vi "HFRR ADV v024 new software.vi"() -> ()   [LabVIEW 2025] (continued)
-:"], ["Ch-Heater:", "НАГРЕВ:"], ["Ch-Humidity Wet:", "CH-Увлажнение:"], ["Ch-Humidity Dry:", "CH-Осушение:"], ["Heater On", "НАГРЕВ ВКЛ"], ["Heater Off", "НАГРЕВ ВЫКЛ"], ["On", "ВКЛ"], ["Off", "ВЫКЛ"], ["TEXT REPORT", "ПРОТОКОЛ ИСПЫТАНИЯ"], ["Open Data File", "ОТКРЫТЬ ФАЙЛ ДАННЫХ"], ["Refresh", "ОБНОВЛЕНО"], ["Tittle", "заглавие"], ["Sample Design", "Образец"], ["Tested date", "Дата"], ["Sample ID ", "Имя образца"], ["Tested by", "Испытано"], ["System Configured Printers ", "Сконфигурированные принтеры"], ["Selected Printer", "Выбранный принтер"], ["Select Printer 3", "Выбрать  Печать"], ["Print", "Печать"], [":-@(WINDUCOM : RECIPROCATORY TEST RIG    DEFINITON FILE )      ", "(Анализатор HFRR с возвратно-поступательным механизмом для определения смазывающей способности дизельных топлив )"], ["Tested by:", "Оператор:"], ["          TIME;      COF;       STROKE  (mm);     AIR TEMP ( Deg C);  TEMP ( Deg C);  HUMIDITY ( Rh );", "КОЭФФИЦИЕНТ ТРЕНИЯ;   Инсульт; ТЕМПЕРАТУРА ВОЗДУХА; ВЛАЖНОСТЬ;"], ["Export", "Экспорт"], ["Temperature Intercept :", "ТЕМП перехват:"], ["Air Temperature Intercept:", "ТЕМП  ВОЗДУХА перехват:"], ["Select File Type ", "Выберете формат файла"], ["S.NO", "S.NO"], ["Trip", ""]]
  out "Residual Uno":string
  out "Residual Due":string
  out "String":string="C:\\Winducom 2010\\1582\\1582\\"
  out "file path":path=path "C:/Windows/wndcm_pw_stdED hfrr.txt"
  out "string":string="49\r50\r51\r10"
  out "x = y?":bool
  out "dipl pwd":string="@143$\n"
  out "string1 4":string
  out "string1 3":string
  out "string1 2":string
  out "string1":string
  out "stopT":bool
  out "Elapsed time 3":dbl=0.10620016403198242 min=0.0 max=6000.0 step=0.01 format="%<%H:%M:%S>t"
  in  "error in (no error)":errorcluster
  out "error out":errorcluster
  in  "RSTCOF 2":bool
  out "PID output":dbl=42.16277107130474 format="%.2f"
  out "Flag":dbl format="%.2f"
  in  "Tab Control 3":enum32{"RMS", "LIVE"}(tab)
  out "array w/ subset deleted":dbl[](array[numeric])
  out "REMARKS":string="@WINDUCOM : RECIPROCATORY TEST RIG    DEFINITON FILE       \r  Sample ID :- , Load :-  2.00 N , Remarks :- , Date :- 05/11/2016, 06:04\r"
  out "Time 2":dbl=0.0004
  in  "reinit":bool=TRUE
  in  "Remarks : 2":string
  out "PID-out":dbl
  out "Rate":dbl=2500.0 caption="Rate (Hz)" min=100.0 max=10000.0 step=1.0
  out "COUNT":i32
  out "FRICVALZ":dbl
  out "Sensor mean 3":dbl
  out "Sensor mean":dbl(slide) min=0.0 max=5.0 step=0.001 scale=0.0..5.0
  out "Sensor mean 2":dbl
  in  "ao0":errorcluster
  out "String 2":string
  out "clk":dbl min=0.0 max=999999999.0 step=0.25 format="%.2f"
  out "spm":string
  out "stp":dbl=0.25 min=0.25 max=60.0 step=0.25 format="%.2f"
  # "© Copyright 2023 | Paltro Inc"
  # "HFRR ADV"
  # "ADV"
  # "Camera Initialization in Progress"
  # "Test Setup"
  # "SAMPLE INFO"
  # "Hz"
  # "grams"
  # "mm"
  # "°C"
  # "%RH"
  # "min"
  # "mins remaining"
  # "°C"
  # "Coefficient of Friction"
  # "Frictional Force ( N )"
  # "Electrical Contact Resistance ( % )"
  # "Temperature ( °C )"
  # "Heater"
  # "( mm )"
  # "Hz"
  # "%Rh"
  # "Stroke ( mm )"
  # "Controller"
  # "%"
  # "N"
  # "deg C"
  # "N"
  # "Automated Scar Detection in Progress"
  # "Zoom Factor"
  # "%"
  # "Tools"
  # "Wear Scar Measurements"
  # "Wear Scar"
  # "Wear Scar"
  # "Wear Scar"
  # "µm"
  # "µm"
  # "µm"
  # "Calibration Centre\nSelect a calibration procedure to begin. Each procedure guides you through all required steps."
  # "Apply known deadweight loads to validate \nthe friction force measurement chain \nand compute the calibration factor for the f\norce transducer."
  # "Step-by-step guided displacement calibration \nacross 6 positions from 0.1 mm to 1.2 mm. Tear \nfirst, then measure each position one by one."
  # "Two-set calibration: one point at 0 °C \nice-point) and one at 60 °C (high-point) \nusing a  reference Calibrator."
  # "Step 1 — Pre-calibration Setup"
  # "Prepare the displacement calibration reference gauge. Ensure the LVDT sensor is connected and the carriage slides freely. You will be guided through 6 positions from 0.2 mm to 1.2 mm, one at a time"
  # "Step 7 — Tare ( ZERO REFERENCE )"
  # "Before measuring, the sensor must be zeroed. Move the carriage to the mechanical zero stop — no displacement applied. Once in position, tap Tare & Begin to zero the reference."
  # "Step 8 — POSITION MEASUREMENT"
  # "Measurement Checklist"
  # "Position the carriage at exactly this \nvalue using your reference gauge, then tap Confirm &\n Next."
  # "All 6 positions recorded!\n\nTap Confirm & Next  to review the calibration summary."
  # "Step 9 — CALIBRATION RESULT"
  # "Stroke Calibration Complete\nAll 6 positions (0.2 mm – 1.2 mm)"
  # "Calibrates the sample/bath temperature sensor. \nUsed for test specimen and lubricant temperature measurement."
  # "Calibrates the ambient air temperature sensor. \nUsed for environmental chamber monitoring."
  # "Set B\n60 °C\nHigh-point calibration"
  # "Set A\n0 °C\nIce-point calibration"
  # "Set B\n60 °C\nHigh-point calibration"
  # "Set A\n0 °C\nIce-point calibration"
  # "Select Temperature Sensor"
  # "Choose which temperature sensor you are calibrating. Both use the same two-\npoint procedure: 0 °C (ice-point) and 60 °C (high-point)."
  # "Step 1 — Reference Instrument Setup"
  # "Connect a calibrated reference to the DUT port. This calibration performs two sets: one at 0 °C and one at 60 °C."
  # "Set A\n0 °C\nIce-point calibration"
  # "Set B\n60 °C\nHigh-point calibration"
  # "Allow the temperature bath to stabilise for at least 2 minutes at each set-point before recording the reading."
  # "Step 2 — Set A:  0 °C Calibration"
  # "Connect the  0 °C reference connector. Wait for the temperature to stabilise. Once stable, and click Record Point."
  # "Step 3 — Set A:  60 °C Calibration"
  # "Connect the  60 °C reference connector. Wait for the temperature to stabilise. Once stable, and click Record Point."
  # "Step 1 — Reference Instrument Setup"
  # "Connect a calibrated reference to the DUT port. This calibration performs two sets: one at 0 °C and one at 60 °C."
  # "Set A\n0 °C\nIce-point calibration"
  # "Set B\n60 °C\nHigh-point calibration"
  # "Allow the temperature bath to stabilise for at least 2 minutes at each set-point before recording the reading."
  # "Step 2 — Set A:  0 °C Calibration"
  # "Connect the  0 °C reference connector. Wait for the temperature to stabilise. Once stable, and click Record Point."
  # "Step 3 — Set A:  60 °C Calibration"
  # "Connect the  60 °C reference connector. Wait for the temperature to stabilise. Once stable, and click Record Point."
  # "System Control Commands\nS;1 - Starts the full automation cycle (Runs Priming-humidify till 70RH sequence first, then switches to Maintenance).\nS;0 - Stops the system immediately and enters Standby mode (Safe State: All actuators OFF).\nM;1 - Skips the priming sequence and jumps directly to Maintenance mode (PID control).\nR;1 - Resets the logic state machine and clears all errors, returning to Standby.\nService Mode (Manual Control)\nX;1 - Enters Manual Service Mode. This disables all automatic logic, sensor safety checks, and timers.\nX;0 - Exits Manual Service Mode and returns to Standby (Safe State).\nActuator Commands (Only work after sending X;1)\nP;[0-255] - Sets the Pump PWM. Note that this is Active Low (0 = Max Flow, 255 = Pump OFF).\nF;I;[0-255] - Sets the Intake Fan speed (0 = OFF, 255 = Max Speed).\nF;O;[0-255] - Sets the Exhaust Fan speed (0 = OFF, 255 = Max Speed).\nD;1 - Turns the Dehumidifier Relay ON.\nD;0 - Turns the Dehumidifier Relay OFF."
  # "%RH"
  # "ISO : WS1.4"
  # "Start test and end test log--- done\nDisable heater ON and Humidity ON during the test --- done\ntemprature and ---done\nhumidity reach log\nauto start run true logic and log\nmanual start log once"
  # "Reference Fluid Information"
  # "Note:\nMake sure to place all images in the folder \"C:\\WinDucom\\im\" before clicking on \"Import Image.\""
  # "NOTE:\nPlace all the images in the path \"C:\\WinDucom\\im\" before clicking on Import Image"
  # "Wear Scar Measurements"
  # "Reference Fluid Information"
  # "Graph :"
types:
  T1 = enum32{"Home", "Dashboard", "Imaging", "Report", "Analysis", "About", "Test Setup", "Advance", "Calibration"}
  T2 = enum32{"HOME", "Test Setup", "Acquire", "Adv Scar", "Adv Scar Report", "Compare Files", "Calibration", "About", "Advance", "Mooha"}
  T3 = enum16{"ASTM D6079", "ISO 12156", "CEC F-096-A-06", "Custom"}
  T4 = enum32{"Dashboard 1", "Dashboard 2", "Dashboard 3"}
  T5 = enum32{"COF", "Friction", "ECR", "Temperature", "Humidity", "Stroke"}
  T6 = enum32{"Coefficient Of Friction", "Air Temperature", "Humidity", "Stroke", "Sample Temperature", "Electrical Contact Resistance", "Frequency", "Air Temp vs Rh"}
  T7 = enum32{"Main", "Stroke", "Friction", "Temperature"}
  T8 = enum32{"Stroke Calibration", "Friction Force Calibration", "Temperature Calibration"}
  T9 = enum32{"Step 1", "Step 2", "Step 3", "Step 4", "Step 5", "Step 6", "Step 7", "Step 8", "Step 9"}
  T10 = enum32{"Test Progress", "Stroke Points Completed"}
  T11 = enum32{"Main", "Step 1", "Step 2", "Step 3", "Air Step 1", "Air Step 2", "Air Step 3"}
  T12 = enum32{"Gains", "Configuration Parameters", "Temperature Calibration"}
  T13 = enum32{"Stroke Data", "Temperature Calibration", "Friction Force Raw Data"}
  T14 = enum32{"COMMUNICATION", "CALIBRATION", "Temp Variables", "Camera", "WO 2465 (1)", "WO 2465 (2)", "WO 2465 (3)"}
  T15 = typedef "Auto Start enum.ctl" = enum16{"Init", "Humidity & Temperature On", "Reach point", "Maintain Stage", "Start Stage", "close", "Exit"}
  T16 = typedef "imagedata.ctl" = cluster{"image type":i32, "image depth":i32, "image":u8[], "mask":u8[], "colors":u32[], "Rectangle":cluster{"left":i16, "top":i16, "right":i16, "bottom":i16}}
  T17 = enum32{"HOME", "Test Setup", "Acquire", "Compare Files", "Print Report", "About", "Advance", "Mooha"}
  T18 = cluster{"Read Heave and Surge":string, "Bytes at Heave Port":dbl, "Heave and Surge COM Port:":refnum<visa-resource-name>, "Com Port 2":refnum<visa-resource-name>, "Residual Due":string, "Heave COM Status 2":bool, "Heave COM Status":bool, "Port 2":bool, "Sway PPR":dbl, "Surge PPR":dbl, "Heave PPR":dbl, "Sway Pitch":dbl, "Surge Pitch":dbl, "Heave Pitch":dbl, "Sway Pulses/mm":dbl, "Surge Pulses/mm":dbl, "Heave Pulses/mm":dbl, "inner loop":dbl, "Read Heave and Surge 2":string, "String 36":string, "Write S":bool, "WriteCC1":string[], "Heave COM Loop":i32, "LastCom":string, "EXIT":bool, "Error Heave":errorcluster}
  T19 = enum8{"Enabled", "Disabled", "Disabled and Grayed Out"}
  T20 = enum32{"HOME", "Test Setup", "Acquire", "Adv Scar", "Adv Scar Report", "Compare Files", "About", "Advance", "Mooha"}
  T21 = enum16{"Always On", "Always Off", "Off While Running"}
  T22 = typedef "POST ANALYSIS ENUM.ctl" = enum16{"OPEN EXE", "INIT", "OPEN FILE", "FIT", "DRAW REC", "DRAW LINE", "PAN", "ZOOM IN", "ZOOM OUT", "SET ZOOM", "CLEAR ROI", "GET MEASUREMENTS", "RESIZE MODE", "STREAM START", "STREAM STOP", "SHOW UI", "MINIMIZE UI", "HIDE UI", "CKISE APP", "CLOSE CONNECTION", "SAVE IMAGE", "SET ROI COLOR", "READ", "TCP CHECK", "CLOSE"}
  T23 = typedef "CAMERA LIVE FEED ENUM.ctl" = enum16{"OPEN EXE", "INIT", "READ", "CAMERA CONNECT", "CAMERA START", "CAMERA STOP", "CAMERA GRAY", "CAMERA RGB", "CAMERA MINIMIZE", "CAMERA CLOSE", "CAMERA MODE LIST", "CAMERA MODE SET", "CAMERA RESTORE", "CAMERA SAVE", "CLOSE"}
  T24 = enum32{"Home", "Dashboard", "Imaging", "Report", "Analysis", "About", "Test Setup", "Advance"}
  T25 = cluster{"File Name":string, "Test Method":string, "Operator":string, "Fuel Description":string, "Date and time":string}
  T26 = enum32{"Home", "Dashboard", "Imaging", "Report", "Analysis", "About", "Test Setup"}
  T27 = enum32{"HOME", "Test Setup", "Acquire", "Compare Files", "About", "Advance", "Mooha"}
  T28 = enum16{"deny read/write", "deny write-only", "deny none"}
  T29 = typedef "NI_ReportGenerationCore.lvlib/HTML Report Image Alignment.ctl" = enum16{"(default)", "LEFT", "RIGHT", "TOP", "TEXTTOP", "MIDDLE", "ABSMIDDLE", "BASELINE", "BOTTOM", "ABSBOTTOM"}
  T30 = enum16{"open", "replace", "create", "open or create", "replace or create", "replace or create with confirmation"}
  T31 = enum16{"INIT", "READ", "MANUAL WRITE", "WRITE", "CLOSE", "ERROR INIT"}
  T32 = enum16{"open", "open or create", "create or replace", "create", "open (read only)"}
  T33 = cluster{"Mode":enum16{"RTU", "ASCII"}, "Slave Address":u8}
diagram:
  w2 = 0.0 ("ch0_filt")
  w4 = -9999999.0 ("max_ch0")
  w5 = 9999999.0 ("min_ch0")
  w17 = FALSE ("Visible")
  w18 = T19."Enabled" ("Disabled")
  w21 = FALSE ("Visible")
  w20 = FALSE ("Humidity Off Command")
  w38 = "" ("USER ID")
  (unwired) T20."HOME" ("Main Tab")
  # "[CH1]    - FF\n[CH2]   - TEMPERATURE\n[CH3]    - Humidity\n[CH4]    - AIR TEMP\n[CH5]\\- Visa Uno\n[CH6] \\- Visa Due\n[CH7]  \\- file path\n[CH8]   - Displacement Gain\n[CHA]   - Stroke Gain\n[CHB]   - Stroke PID Gain\n[CHC]   -Language Selection\n[CHD]   -Power +\n[CHE]   -Power_\n[CHF]   -Heater\n[CHG]   -Humidity Wet\n[CHH]   -Humidity Dry\n[CHI]   -Integral Time \n[CHIJ   -Air intercept\n[CHI]   -Temp Intercept"
  n1 = flat-sequence {
    tunnel: [w62] -> w1
    tunnel: w1 -> [_]
    tunnel: [w108] -> w30
    tunnel: w30 -> [w122]
    tunnel: [w121] -> w29
    tunnel: ["ao0"] -> w32
    tunnel: w29 -> [_]
    tunnel: w32 -> [w186]
    tunnel: [w186] -> w31
    tunnel: w31 -> [w227]
    tunnel: [w225] -> w42
    tunnel: [w227] -> w41
    tunnel: w42 -> [w277]
    tunnel: w41 -> [w234]
    tunnel: [w277] -> w28
    tunnel: [w240] -> w27
    tunnel: [w228] -> w26
    tunnel: [w283] -> _
    tunnel: [w282] -> _
    tunnel: [w284] -> w61
    tunnel: w28 -> [w284]
    tunnel: w27 -> [w282]
    tunnel: w26 -> [w283]
    frame #0 {
      n2 = call "Read Config.vi"() -> ("error out"=w62:errorcluster, "STROKE PARAMETERS"=w67:dbl[], "ADC PARAMETERS"=w68:dbl[], "PID  PARAMETERS"=w69:dbl[], "Stroke Calibration"=w66:string)  [unwired: 7 in]
      n3 = Index Array(array=w69) -> (element #1=w71:dbl, element #2=w72:dbl, element #3=w73:dbl, element #4=w74:dbl, element #5=w75:dbl, element #6=w76:dbl, element #7=w77:dbl, element #8=w78:dbl, element #9=w79:dbl)  [unwired: 9 in]
      n4 = Index Array(array=w68) -> (element #1=w80:dbl, element #2=w81:dbl, element #3=w82:dbl, element #4=w83:dbl)  [unwired: 4 in]
      n5 = Index Array(array=w67) -> (element #1=w84:dbl, element #2=w85:dbl)  [unwired: 2 in]
      n6 = Spreadsheet String To Array(delimiter (Tab)=";", format string="", spreadsheet string=w66, array type (2D Dbl)=dbl[] []) -> (array=w70:dbl[])
      n7 = local write "VREF"(w80) -> ()
      n8 = local write "ADC_Resolution"(w81) -> ()
      n9 = local write "PIEZO_CAL_FACTOR"(w82) -> ()
      n10 = local write "NORMAL_FORCE"(w83) -> ()
      n11 = local write "STROKE FILTER"(w84) -> ()
      n12 = local write "Add up Stroke"(w85) -> ()
      n13 = local write "calibration values"(w70) -> ()
      n14 = local write "milliseconds to wait"(w71) -> ()
      n15 = local write "dt"(w72) -> ()
      n16 = local write "kp"(w73) -> ()
      n17 = local write "ki"(w74) -> ()
      n18 = local write "kd"(w75) -> ()
      n19 = local write "max_step_change"(w76) -> ()
      n20 = local write "max_amplitude"(w77) -> ()
      n21 = local write "min_amplitude"(w78) -> ()
      n22 = local write "startup_cmd"(w79) -> ()
    }
    frame #1 {
      n23 = disable-structure shown="Disabled" {
        frame Disabled {
          n24 = control-ref of="This VI"() -> (w96:refnum<vi>)
          n25 = property class="VI"(reference=w96) -> (reference out=w87:refnum<vi>, error out=w91:errorcluster, "Panel"=w95:refnum<vi>)  [unwired: 1 in]
          n26 = property class="Pnl"(reference=w95, error in=w91) -> (reference out=w89:refnum<vi>, error out=w92:errorcluster, "Panes[]"=w94:refnum<vi>[])
          n27 = for {
            tunnel: w94 -> [w102] mode=indexing
            tunnel: T21."Always Off" ("Horizontal Scrollbar Visibility") -> [w101]
            tunnel: w92 -> [w98]
            tunnel: [w97] -> w90
            n28 = property class="Pane"(reference=w102, error in=w98, "HorizScrollbarVisibility"=w101) -> (reference out=w99:refnum<vi>, error out=w100:errorcluster)
            n29 = Close Reference(reference=w99, error in (no error)=w100) -> (error out=w97:errorcluster)
          }
          n30 = Close Reference(reference=w89, error in (no error)=w90) -> (error out=w88:errorcluster)
          n31 = Close Reference(reference=w87, error in (no error)=w88) -> (error out=→"error out 8":errorcluster)
        }
        frame Enabled {
        }
      }
    }
    frame #2 {
      n32 = call "CLOSE CONNECTION.vi"("error in (no error)"="error in (no error) 2") -> ("error out"=w106:errorcluster)  [unwired: 10 in]
      n33 = call <vilib>:"Clear Errors.vi"("error in (no error)"=w106) -> ("error out"=w105:errorcluster)  [unwired: 5 in, 1 out]
      n34 = disable-structure shown="Enabled" {
        disable-tunnel: w105 -> [w112 _]
        disable-tunnel: [w111 _] -> w108
        frame Enabled {
          n35 = call <userlib>:"Fit VI window to Largest Dec.vi"("error in (no error)"=w112, "border spacing (2 px)"=1) -> ("error out"=w115:errorcluster, "dup VI Ref"=w119:refnum<vi>)  [unwired: 4 in]
          n36 = invoke on="Invoke Node" class="VI" method="FP.Run-Time Position.Maximized"(reference=w119, error in=w115) -> (error out=w116:errorcluster)  [unwired: 2 in, 3 out]
          n37 = call <vilib>:"Clear Errors.vi"("error in (no error)"=w116) -> ("error out"=w118:errorcluster)  [unwired: 5 in, 1 out]
          n38 = control-ref of="This VI"() -> (w110:refnum<vi>)
          n39 = invoke on="Invoke Node" class="VI" method="Default Vals.Reinit All"(reference=w110, error in=w118) -> (reference out=w114:refnum<vi>, error out=w113:errorcluster)  [unwired: 1 in, 1 out]
          n40 = Close Reference(reference=w114, error in (no error)=w113) -> (error out=w111:errorcluster)
        }
        frame Disabled {
        }
      }
      n41 = local write "sign in temp"(FALSE ("sign in temp")) -> ()
      n42 = property on="Sign In" class="Bool (strict)"("DisabledEnum"=T19."Disabled" ("Disabled")) -> ()  [unwired: 2 in, 2 out]
      n43 = property on="Auto Scar Check" class="Clust (strict)"("Visible"=TRUE) -> ()  [unwired: 2 in, 2 out]
    }
    frame #3 {
      n44 = call "dialog box.vi"("Status"="Before starting the test, verify that the microscope cable is connected.", "error in"=w122) -> ("error out"=w121:errorcluster)  [unwired: 8 in]
    }
    frame #4 {
      (unwired) TRUE ("Re-Initialise")
      w128 = FALSE ("Upld AR 2")
      # "kkkkk"
      # "C:\\Windows\\wndcm_pw_stdED hfrr.txt"
      # "C:\\LAB-IQ NXT"
      # "C:\\LAB-IQ NXT\\wndcm_pw_stdED hfrr.txt"
      # "password file"
      n45 = Current VI's Path() -> (path=w141:path)
      n46 = Strip Path(path=w141) -> (stripped path=w134:path)  [unwired: 1 out]
      n47 = Path To String(path=w134) -> (string=w136:string)
      n48 = local write "conststatus"(0.0 ("rpm value : 2")) -> ()
      n49 = local write "Upld AR 2"(TRUE ("Upld AR 2")) -> ()
      n50 = local write "Lan flag"(0.0 ("Lan flag")) -> ()
      n51 = local write "COUNT"(0 ("COUNT")) -> ()
      n52 = local write "FLAG 2"(0.0 ("FLAG 2")) -> ()
      n53 = local write "Com flag"(u32 0 ("Com flag")) -> ()
      n54 = local write "refresh flag"(FALSE ("refresh flag")) -> ()
      n55 = local write "Json St Flg"(w128) -> ()
      n56 = Search/Split String(string=w136, search string/char (-)=".exe") -> (match + rest of string=w138:string)  [unwired: 1 in, 2 out]
      n57 = Match True/False String(2:".vi" ("false string"), 3:".exe" ("true string"), 4:w138) -> (0:w135:bool)  [unwired: 1 out]
      n58 = local write "Json End Flg"(w128) -> ()
      n59 = case shown="True" w135 {
        tunnel: w134 -> [w157 w159]
        tunnel: [w157 w158] -> w132
        frame False {
        }
        frame True {
          n60 = Strip Path(path=w159) -> (stripped path=w158:path)  [unwired: 1 out]
        }
      }
      n61 = Path To String(path=w132) -> (string=→"Gain path":string)
      n62 = local write "Main Tab Display"(T4."Dashboard 1" ("Main Tab Display")) -> ()
      n63 = local write "main tab sub"(enum32{"Page 1", "Page 2"}."Page 1" ("main tab sub")) -> ()
      n64 = local write "Main Tab"(T2."HOME" ("Main Tab")) -> ()
      n65 = local write "EVENT LOG"("") -> ()
      n66 = List Folder(path=path "C:/LAB-IQ" ("directory path"), pattern="*.txt") -> (filenames=w147:string[])  [unwired: 2 in, 3 out]
      n67 = Search 1D Array(1D array=w147, element="wndcm_pw_stdED hfrr.txt") -> (index of element=w150:i32)  [unwired: 1 in]
      n68 = Equal?(x=w150, y=-1) -> (x = y?=w145:bool)
      n69 = case shown="True" w145 {
        frame False {
        }
        frame True {
          n70 = String To Byte Array(string="123\n") -> (unsigned byte array=w164:u8[])
          n71 = Array Size(array=w164) -> (size(s)=w163:i32)
          n72 = for {
            N: w163 -> [_]
            tunnel: w164 -> [w177]
            tunnel: [w174] -> w166 mode=indexing
            tunnel: w163 -> [w169]
            i -> [w167]
            n73 = Decrement(x=w169) -> (x-1=w170:i32)
            n74 = Equal?(x=w167, y=w170) -> (x = y?=w171:bool)
            n75 = Index Array(array=w177, index=w167) -> (element=w176:u8)
            n76 = Number To Decimal String(number=w176) -> (decimal integer string=w175:string)  [unwired: 1 in]
            n77 = Select(t="", s=w171, f="\r") -> (s? t:f=w168:string)
            n78 = Concatenate Strings(w175, w168) -> (w174:string)
          }
          n79 = local read "file path"() -> (w160:path)
          n80 = Concatenate Strings(w166) -> (w162:string)
          n81 = call <vilib>:"Write Characters To File.vi"("append to file? (new file:F)"=FALSE, "character string"=w162, "file path (dialog if empty)"=w160) -> ()  [unwired: 2 in, 1 out]
        }
      }
      n82 = local write "clk"(0.0 ("clk")) -> ()
      n83 = local write "Flag"(0.0 ("Flag")) -> ()
      "file path" <- path "C:/LAB-IQ/wndcm_pw_stdED hfrr.txt" ("file path")
      "FF buffer" <- dbl[] [] ("FF buffer")
    }
    frame #5 {
      # "C:\\WinDucom\\calibrate WO 2391.dcf"
      n84 = String To Path(string="C:\\LAB-IQ\\calibrate WO 2465.dcf") -> (path=w185:path)
      n85 = Open/Create/Replace File "Open File"(file path (use dialog)=w185) -> (refnum out=w184:refnum<file>)  [unwired: 5 in, 2 out]
      n86 = for {
        N: 24 -> [_]
        tunnel: w184 -> [w205]
        i -> [w199]
        (unwired) TRUE ("line mode (F)")
        n87 = Read from Text File "Read File"(file (use dialog)=w205) -> (text=w204:string)  [unwired: 3 in, 3 out]
        n88 = Match Pattern(string=w204, regular expression="]") -> (after substring=w202:string)  [unwired: 1 in, 3 out]
        n89 = String Subset(string=w204, offset (0)=5, length (rest)=10 ("length (rest)")) -> (substring=w197:string)
        n90 = Fract/Exp String To Number(string=w197) -> (number=w198:dbl)  [unwired: 3 in, 1 out]
        n91 = Match Pattern(string=w202, regular expression="-") -> (before substring=w200:string)  [unwired: 1 in, 3 out]
        n92 = case shown="15" w199 {
          tunnel: w198 -> [w208 w209 w210 w211 _ _ _ w216 w217 _ w218 _ _ _ _ _ _ w219 w220 _ _ _ _ _ _]
          tunnel: w200 -> [_ _ _ _ w212 w213 w214 _ _ _ _ _ _ _ _ _ _ _ _ w221 w222 _ w223 w224 _]
          frame 0 {
            n93 = local write "FRIC. FORCE :"(w208) -> ()
          }
          frame 1 {
            n94 = local write "TEMPERATURE :"(w209) -> ()
          }
          frame 2 {
            n95 = local write "HUMIDITY:"(w210) -> ()
          }
          frame 3 {
            n96 = local write "AIR TEMPERATURE :"(w211) -> ()
          }
          frame 4 {
            n97 = local write "Com Port 1"(w212) -> ()
          }
          frame 5 {
            n98 = local write "Com Port 2"(w213) -> ()
            n99 = local write "visa due"(w213) -> ()
          }
          frame 6 {
            n100 = String To Path(string=w214) -> (path=w215:path)
            n101 = local write "File Path"(w215) -> ()
          }
          frame 7 {
            n102 = local write "DISPLACEMENT :"(w216) -> ()
          }
          frame 8 {
            n103 = local write "STROKE GAIN :"(w217) -> ()
          }
          frame 9 {
          }
          frame 10 {
            n104 = local write "Language Selection"(w218) -> ()
          }
          frame 11 {
          }
          frame 12 {
          }
          frame 13 {
          }
          frame 14 {
          }
          frame 15 {
          }
          frame 16 {
          }
          frame 17 {
            n105 = local write "AIR TEMP INTERCEPT:"(w219) -> ()
          }
          frame 18 {
            n106 = local write "TEMP INTERCEPT:"(w220) -> ()
          }
          frame 21 {
            n107 = local write "S.NO"(w221) -> ()
          }
          frame 22 {
            n108 = local write "Com Port 3"(w222) -> ()
          }
          frame 23 {
          }
          frame 19 {
            n109 = local write "C3 :"(w223) -> ()
          }
          frame 20 {
            n110 = local write "Camera Port :"(w224) -> ()
          }
          frame 24, Default {
          }
        }
      }
      n111 = String To Path(string="C:\\LAB-IQ\\Image Calibrate v01.dcf") -> (path=w181:path)
      n112 = Open/Create/Replace File ("Open File")(file path (use dialog)=w181) -> (refnum out=w180:refnum<file>)  [unwired: 5 in, 2 out]
      n113 = for {
        N: 4 -> [_]
        tunnel: w180 -> [w192]
        i -> [w188]
        n114 = Read from Text File ("Read File")(file (use dialog)=w192) -> (text=w193:string)  [unwired: 3 in, 3 out]
        n115 = String Subset(string=w193, offset (0)=6, length (rest)=10 ("length (rest)")) -> (substring=w189:string)
        n116 = Fract/Exp String To Number(string=w189) -> (number=w187:dbl)  [unwired: 3 in, 1 out]
        n117 = case shown="3" w188 {
          tunnel: w187 -> [w194 w195 _ w196 _]
          frame 0 {
            n118 = local write "5x Gain"(w194) -> ()
          }
          frame 1 {
            n119 = local write "10x Gain"(w195) -> ()
          }
          frame 2 {
          }
          frame 3 {
            n120 = local write "100x gain"(w196) -> ()
          }
          frame 4, Default {
          }
        }
      }
    }
    frame #6 {
      n121 = Wait (ms)(milliseconds to wait=u32 1000) -> (millisecond timer value=w225:u32)
    }
    frame #7 {
      w243 = u32 2000 ("milliseconds to wait")
      w270 = u32 2000 ("milliseconds to wait")
      n122 = call "CAMERA LIVE FEED FGV.vi"("Enum - Menu"=CAMERA_LIVE_FEED_ENUM."OPEN EXE", "error in (no error)"=w234) -> ("error out"=w276:errorcluster)  [unwired: 8 in, 1 out]
      n123 = call "Stall Data Flow.vim"("value in"=w276, "milliseconds to wait"=w270) -> ("value out"=w274:errorcluster)  [unwired: 1 out]
      n124 = call "CAMERA LIVE FEED FGV.vi"("Enum - Menu"=CAMERA_LIVE_FEED_ENUM."INIT", "error in (no error)"=w274) -> ("error out"=w272:errorcluster)  [unwired: 8 in, 1 out]
      n125 = call "IMAGE ANALYSIS.vi"("Enum"=POST_ANALYSIS_ENUM."OPEN EXE", "error in"=w234) -> ("error out"=w231:errorcluster)  [unwired: 8 in, 1 out]
      n126 = case shown="Error .." w272 {
        selector: w272 -> [w278 _]
        tunnel: [w278 _] -> w271
        frame No Error {
        }
        frame Error {
          n127 = One Button Dialog(message="Camera initialization error.\nPlease Restart the software") -> ()  [unwired: 1 in, 1 out]
        }
      }
      n128 = call "Stall Data Flow.vim"("value in"=w231, "milliseconds to wait"=u32 8000) -> ("value out"=w230:errorcluster)  [unwired: 1 out]
      n129 = property on="Camera Port :" class="CmbBox"() -> ("Strings[]"=w268:string[], "Value"=w269:string)  [unwired: 2 in, 2 out]
      n130 = call "IMAGE ANALYSIS.vi"("Enum"=POST_ANALYSIS_ENUM."INIT", "error in"=w230) -> ("error out"=w228:errorcluster)  [unwired: 8 in, 1 out]
      n131 = Search 1D Array(1D array=w268, element=w269) -> (index of element=w267:i32)  [unwired: 1 in]
      n132 = Type Cast(type=30, x=w267) -> (*(type *) &x=w265:i32)
      n133 = call "Stall Data Flow.vim"("value in"=w271, "milliseconds to wait"=w270) -> ("value out"=w247:errorcluster)  [unwired: 1 out]
      n134 = Add(x=w265, y=48) -> (x+y=w246:i32)
      n135 = call "CAMERA LIVE FEED FGV.vi"("Enum - Menu"=CAMERA_LIVE_FEED_ENUM."CAMERA CONNECT", "error in (no error)"=w247, "CAMERA PORT"=w246) -> ("error out"=w256:errorcluster)  [unwired: 7 in, 1 out]
      n136 = call "Stall Data Flow.vim"("value in"=w256, "milliseconds to wait"=u32 5000) -> ("value out"=w257:errorcluster)  [unwired: 1 out]
      n137 = call "CAMERA LIVE FEED FGV.vi"("Enum - Menu"=CAMERA_LIVE_FEED_ENUM."CAMERA MODE LIST", "error in (no error)"=w257) -> ("error out"=w259:errorcluster)  [unwired: 8 in, 1 out]
      n138 = call "Stall Data Flow.vim"("value in"=w259, "milliseconds to wait"=w243) -> ("value out"=w258:errorcluster)  [unwired: 1 out]
      n139 = call "CAMERA LIVE FEED FGV.vi"("Enum - Menu"=CAMERA_LIVE_FEED_ENUM."READ", "error in (no error)"=w258) -> ("error out"=w245:errorcluster, "data out"=→"Camera List":string)  [unwired: 8 in]
      n140 = call "Stall Data Flow.vim"("value in"=w245, "milliseconds to wait"=w243) -> ("value out"=w244:errorcluster)  [unwired: 1 out]
      n141 = Type Cast(type=30, x=0) -> (*(type *) &x=w239:i32)
      n142 = Add(x=w239, y=48) -> (x+y=w237:i32)
      n143 = call "CAMERA LIVE FEED FGV.vi"("Enum - Menu"=CAMERA_LIVE_FEED_ENUM."CAMERA MODE SET", "error in (no error)"=w244, "CAMERA MODE"=w237) -> ("error out"=w241:errorcluster)  [unwired: 7 in, 1 out]
      n144 = call "Stall Data Flow.vim"("value in"=w241, "milliseconds to wait"=u32 2000) -> ("value out"=w261:errorcluster)  [unwired: 1 out]
      n145 = call "CAMERA LIVE FEED FGV.vi"("Enum - Menu"=CAMERA_LIVE_FEED_ENUM."CAMERA START", "error in (no error)"=w261) -> ("error out"=w262:errorcluster)  [unwired: 8 in, 1 out]
      n146 = call "Stall Data Flow.vim"("value in"=w262, "milliseconds to wait"=u32 1000) -> ("value out"=w263:errorcluster)  [unwired: 1 out]
      n147 = call "CAMERA LIVE FEED FGV.vi"("Enum - Menu"=CAMERA_LIVE_FEED_ENUM."CAMERA MINIMIZE", "error in (no error)"=w263) -> ("error out"=w240:errorcluster)  [unwired: 8 in, 1 out]
    }
    frame #8 {
      n148 = case shown="No Error" w282 {
        frame No Error {
          n149 = property on="Auto Scar Check" class="Clust (strict)"("Visible"=FALSE) -> ()  [unwired: 2 in, 2 out]
        }
        frame Error {
        }
      }
      n150 = local write "sign in temp"(TRUE ("sign in temp")) -> ()
      n151 = property on="Sign In" class="Bool (strict)"("DisabledEnum"=T19."Enabled" ("Disabled")) -> ()  [unwired: 2 in, 2 out]
    }
  }
  n152 = local write "Cal Password"("" ("Cal Password")) -> ()
  n153 = property on="Auto Start Test" class="Bool (strict)"("Visible"=TRUE) -> ()  [unwired: 2 in, 2 out]
  n154 = property on="FRICVALZ 2" class="Bool (strict)"("DisabledEnum"=w18) -> ()  [unwired: 2 in, 2 out]
  n155 = property on="FRICVALZ 4" class="Bool (strict)"("DisabledEnum"=w18) -> ()  [unwired: 2 in, 2 out]
  n156 = property on="FRICVALZ 3" class="Bool (strict)"("DisabledEnum"=w18) -> ()  [unwired: 2 in, 2 out]
  n157 = property on="About" class="Clust (strict)"("Visible"=FALSE) -> ()  [unwired: 2 in, 2 out]
  n158 = property on="Tab Control 5" class="TabCtl (strict)"("Tabs Visible?"=TRUE ("Page Labels Display Visible?")) -> ()  [unwired: 2 in, 2 out]
  n159 = property on="Wrong Password" class="Str"("Visible"=w17) -> ()  [unwired: 2 in, 2 out]
  n160 = property on="Calibration 2" class="TabCtl (strict)"("Visible"=w17) -> ()  [unwired: 2 in, 2 out]
  n161 = local write "SCAR MEASURMENT"(enum32{"Auto Scar", "Manual Scar"}."Manual Scar" ("SCAR MEASURMENT")) -> ()
  n162 = local write "Temperature Off Command"(w20) -> ()
  n163 = local write "Main Dashboard Buttons"(T1."Home" ("Main Dashboard Buttons")) -> ()
  n164 = local write "Humidity Off Command"(w20) -> ()
  n165 = local write "CAMERA ROI MIN TEMP"(w20) -> ()
  n166 = local write "TEST FILE NAM,E SAVED"(w20) -> ()
  n167 = local write "LIVE FEED MIN TEMP"(w20) -> ()
  n168 = local write "SCAR MEASURMENT"(enum32{"Auto Scar", "Manual Scar"}."Manual Scar" ("SCAR MEASURMENT")) -> ()
  n169 = local write "Auto stop temp"(w21) -> ()
  n170 = local write "main tab sub"(enum32{"Page 1", "Page 2"}."Page 1" ("main tab sub")) -> ()
  n171 = local write "USERNAME"(w38) -> ()
  n172 = local write "Main Tab"(T2."HOME" ("Main Tab")) -> ()
  n173 = local write "USER ID"(w38) -> ()
  n174 = property on="Auto Scar Check  2" class="Clust (strict)"("Visible"=w21) -> (error out=w24:errorcluster)  [unwired: 2 in, 1 out]
  n175 = property on="Quit" class="Bool (strict)"("Value"=FALSE ("Quit")) -> (error out=w40:errorcluster)  [unwired: 2 in, 1 out]
  n176 = while {
    stop <- w286 stop-if-true
    n177 = event shown="[8] \"Password 3.Service Password\": Value Change" {
      selector: _ -> [_ _ _ _ _ _ _ _ _ _ _ _ _ _ _ _ _ _ _ _ _ _ _ _ _ _ _ _ _ _ _ _ _ _ _ _ _ _ _]
      dyn-events: _ -> [_ _ _ _ _ _ _ _ _ _ _ _ _ _ _ _ _ _ _ _ _ _ _ _ _ _ _ _ _ _ _ _ _ _ _ _ _ _ _]
      timeout: 100 -> [_ _ _ _ _ _ _ _ _ _ _ _ _ _ _ _ _ _ _ _ _ _ _ _ _ _ _ _ _ _ _ _ _ _ _ _ _ _ _]
      tunnel: [FALSE FALSE _ FALSE _ _ _ _ _ _ _ _ _ _ _ _ _ _ _ _ _ _ _ _ _ _ _ _ _ _ _ _ _ _ _ _ _ _ TRUE] -> w286
      event Timeout {
        n178 = event-data() -> ()  [unwired: 1 in, 3 out]
        n179 = disable-structure shown="Disabled" {
          frame Disabled {
            n180 = local read "Auto Start Test"() -> (w300:bool)
            n181 = local read "RUN"() -> (w301:bool)
            n182 = Or(x=w301, y=w300) -> (x .or. y?=w299:bool)
            n183 = case shown="True" w299 {
              frame False {
                w302 = TRUE ("PAUSE")
                n184 = call "ELAPSED TIMER VI - abort test.vi"("RESET"=w302, "PAUSE"=w302) -> ()  [unwired: 7 in, 3 out]
              }
              frame True {
                n185 = local read "Stroke 2"() -> (w307:dbl)
                n186 = local read "FF 3"() -> (w309:dbl)
                n187 = Equal?(x=w307, y=0.95 ("Stroke 2")) -> (x = y?=w304:bool)
                n188 = Equal?(x=w309, y=0.0 ("FF 3")) -> (x = y?=w305:bool)
                n189 = Or(x=w305, y=w304) -> (x .or. y?=w303:bool)
                n190 = case shown="True" w303 {
                  selector: w303 -> [_ w314]
                  frame False {
                    w310 = TRUE ("PAUSE")
                    n191 = call "ELAPSED TIMER VI - abort test.vi"("RESET"=w310, "PAUSE"=w310) -> ()  [unwired: 7 in, 3 out]
                  }
                  frame True {
                    n192 = Not(x=w314) -> (.not. x?=w313:bool)
                    n193 = call "ELAPSED TIMER VI - abort test.vi"("TARGET"=60.0, "RESET"=w313, "PAUSE"=FALSE) -> ("ELAPSED INDICATION"=w311:bool)  [unwired: 6 in, 2 out]
                    n194 = case shown="True" w311 {
                      frame False {
                      }
                      frame True {
                        n195 = stacked-sequence {
                          frame #0 {
                            w316 = FALSE
                            n196 = local write "RUN"(w316) -> ()
                            n197 = local write "Auto Start Test"(w316) -> ()
                          }
                          frame #1 {
                            n198 = One Button Dialog(message="Test stopped due to a communication error. Reconnect the C1 and C2 cables.") -> ()  [unwired: 1 in, 1 out]
                          }
                        }
                      }
                    }
                  }
                }
              }
            }
          }
          frame Enabled {
          }
        }
        n199 = Get Date/Time In Seconds() -> (seconds since 1Jan1904=w297:timestamp)
        n200 = Format Into String(format string="%<%I:%M:%S:%p %d:%B:%Y>T", w297) -> (resulting string=→"Time Stamp":string)  [unwired: 2 in, 1 out]
        n201 = local read "Service Password enable"() -> (w289:bool)
        n202 = local read "FILE"() -> (w294:string)
        n203 = call <vilib>:"Trim Whitespace.vi"("string"=w294) -> ("trimmed string"=w293:string)  [unwired: 1 in]
        n204 = String Length(string=w293) -> (length=w292:i32)
        n205 = Greater?(x=w292, y=1) -> (0:w290:bool)
        n206 = case shown="False" w290 {
          tunnel: w289 -> [w318 _]
          frame False {
            n207 = case shown="False" w318 {
              frame True {
                w319 = "Test Start In Service Mode" ("Tip Strip")
                w320 = T19."Enabled" ("Disabled")
                n208 = property on="Auto Start Test" class="Bool (strict)"("DisabledEnum"=w320, "TipStrip"=w319) -> ()  [unwired: 2 in, 2 out]
                n209 = property on="RUN" class="Bool (strict)"("DisabledEnum"=w320, "TipStrip"=w319) -> ()  [unwired: 2 in, 2 out]
              }
              frame False {
                w321 = "Enter File Name to Start Test" ("Tip Strip")
                w322 = T19."Disabled and Grayed Out" ("Disabled")
                n210 = property on="Auto Start Test" class="Bool (strict)"("DisabledEnum"=w322, "TipStrip"=w321) -> ()  [unwired: 2 in, 2 out]
                n211 = property on="RUN" class="Bool (strict)"("DisabledEnum"=w322, "TipStrip"=w321) -> ()  [unwired: 2 in, 2 out]
              }
            }
          }
          frame True {
            w323 = "" ("Tip Strip")
            w324 = T19."Enabled" ("Disabled")
            n212 = property on="Auto Start Test" class="Bool (strict)"("DisabledEnum"=w324, "TipStrip"=w323) -> ()  [unwired: 2 in, 2 out]
            n213 = property on="RUN" class="Bool (strict)"("DisabledEnum"=w324, "TipStrip"=w323) -> ()  [unwired: 2 in, 2 out]
          }
        }
      }
      event "RUN": Value Change {
        n214 = event-data() -> ()  [unwired: 1 in, 6 out]
        n215 = local read "RUN"() -> (w326:bool)
        n216 = case shown="False" w326 {
          frame False {
            n217 = flat-sequence {
              frame #0 {
                n218 = local write "START TEMP"(FALSE ("START TEMP")) -> ()
              }
              frame #1 {
                n219 = Wait (ms)(milliseconds to wait=u32 1500) -> ()  [unwired: 1 out]
              }
              frame #2 {
              }
              frame #3 {
                n220 = local write "Due Write"("VC;0") -> ()
              }
              frame #4 {
                n221 = Wait (ms)(milliseconds to wait=u32 1500) -> ()  [unwired: 1 out]
              }
              frame #5 {
                w335 = T19."Enabled" ("Disabled")
                (unwired) T24."Imaging" ("Main Dashboard Buttons")
                (unwired) T20."Adv Scar" ("Main Tab")
                w337 = "" ("FILE")
                n222 = local write "measured_stroke"(0.0 ("measured_stroke")) -> ()
                n223 = local write "Due Write"("VC;0") -> ()
                n224 = local write "FILE"(w337) -> ()
                n225 = local write "Batch Ref Num :"(w337) -> ()
                n226 = local write "Fuel Discription :"(w337) -> ()
                n227 = local write "Main Tab"(T2."Adv Scar" ("Main Tab")) -> ()
                n228 = local write "Remarks :"(w337) -> ()
                n229 = local write "Main Dashboard Buttons"(T1."Imaging" ("Main Dashboard Buttons")) -> ()
                n230 = local write "TEST FILE NAM,E SAVED"(FALSE ("TEST FILE NAM,E SAVED")) -> ()
                n231 = property on="Stroke ( mm )" class="WFChart (strict)"("History Data"=cluster{"y":dbl, dbl, "y":dbl}[] []) -> ()  [unwired: 2 in, 2 out]
                n232 = property on="Auto Start Test" class="Bool (strict)"("Visible"=TRUE) -> ()  [unwired: 2 in, 2 out]
                n233 = property on="FRICVALZ 2" class="Bool (strict)"("DisabledEnum"=w335) -> ()  [unwired: 2 in, 2 out]
                n234 = property on="FRICVALZ 4" class="Bool (strict)"("DisabledEnum"=w335) -> ()  [unwired: 2 in, 2 out]
                n235 = property on="FRICVALZ 3" class="Bool (strict)"("DisabledEnum"=w335) -> ()  [unwired: 2 in, 2 out]
              }
            }
          }
          frame True {
            n236 = flat-sequence {
              frame #0 {
                n237 = local write "Due Write"("VC;1") -> ()
              }
              frame #1 {
                n238 = Wait (ms)(milliseconds to wait=u32 2000) -> ()  [unwired: 1 out]
              }
              frame #2 {
                n239 = local write "Due Write"("VC;1") -> ()
              }
              frame #3 {
                n240 = Wait (ms)(milliseconds to wait=u32 2000) -> ()  [unwired: 1 out]
              }
              frame #4 {
                w345 = T19."Disabled" ("Disabled")
                n241 = property on="Auto Start Test" class="Bool (strict)"("Visible"=FALSE) -> ()  [unwired: 2 in, 2 out]
                n242 = local write "START TEMP"(TRUE ("START TEMP")) -> ()
                n243 = property on="FRICVALZ 2" class="Bool (strict)"("DisabledEnum"=w345) -> ()  [unwired: 2 in, 2 out]
                n244 = property on="FRICVALZ 4" class="Bool (strict)"("DisabledEnum"=w345) -> ()  [unwired: 2 in, 2 out]
                n245 = property on="FRICVALZ 3" class="Bool (strict)"("DisabledEnum"=w345) -> ()  [unwired: 2 in, 2 out]
              }
            }
          }
        }
      }
      event "Auto": Value Change {
        n246 = event-data() -> ()  [unwired: 1 in, 6 out]
        n247 = stacked-sequence {
          frame #0 {
            n248 = local write "FILE"("") -> ()
          }
          frame #1 {
            n249 = Get Date/Time In Seconds() -> (seconds since 1Jan1904=w351:timestamp)
            n250 = Format Into String(format string="%<%I_%M_%S_%p_%d_%B_%Y>T", w351) -> (resulting string=w350:string)  [unwired: 2 in, 1 out]
            n251 = local write "FILE"(w350) -> ()
          }
        }
        n252 = local read "Auto"() -> (w348:bool)
        n253 = Not(x=w348) -> (.not. x?=w347:bool)
        n254 = local write "Auto"(w347) -> ()
      }
      event "Auto Start Temp": Value Change {
        n255 = event-data() -> ()  [unwired: 1 in, 6 out]
        n256 = local read "Auto Start Test"() -> (w354:bool)
        n257 = case shown="False" w354 {
          frame False {
            n258 = stacked-sequence {
              frame #0 {
                n259 = local write "START TEMP"(FALSE ("START TEMP")) -> ()
              }
              frame #1 {
                n260 = Wait (ms)(milliseconds to wait=u32 2000) -> ()  [unwired: 1 out]
              }
              frame #2 {
                n261 = local write "Due Write"("VC;0") -> ()
              }
              frame #3 {
                n262 = Wait (ms)(milliseconds to wait=u32 2000) -> ()  [unwired: 1 out]
              }
              frame #4 {
                w364 = T19."Enabled" ("Disabled")
                (unwired) T24."Imaging" ("Main Dashboard Buttons")
                w365 = "" ("FILE")
                n263 = local write "Main Tab"(T2."Adv Scar" ("Main Tab")) -> ()
